vi "python analysis.vi"() -> ()   [LabVIEW 2020, in "Point Grey Camera.lvclass"]
uses:
  Point Grey Camera.lvclass
  Point Grey Camera.lvclass/Point Grey Camera.ctl
panel:
  out "analysis time":u32
  out "FakeCamera out":refnum<class "Point Grey Camera.lvclass">
  in  "FakeCamera in":refnum<class "Point Grey Camera.lvclass">
  out "error out":errorcluster
  in  "error in (no error)":errorcluster
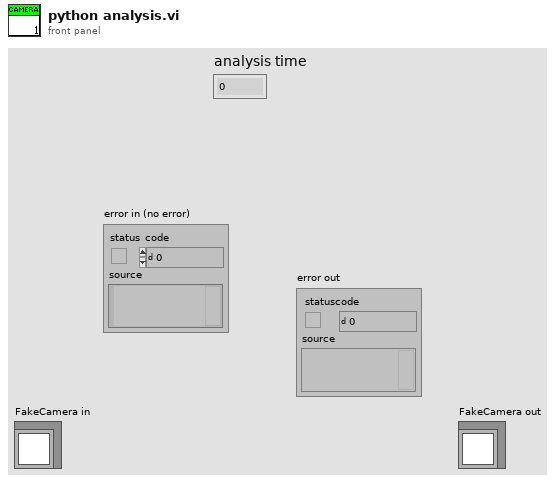
[diagram p1: front panel]
types:
  T1 = typedef "OnOffTypeDef.ctl" = enum16{"off", "on"}
  T2 = typedef "IMAQ Image.ctl" = refnum<image>
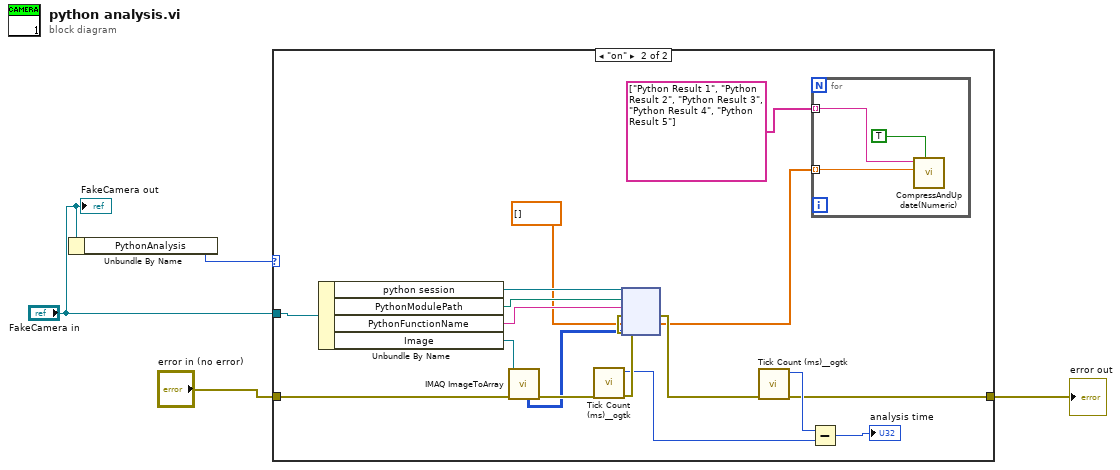
[diagram p0: block diagram]
diagram:
  n1 = Unbundle By Name("FakeCamera in") -> ("PythonAnalysis"=w1:T1)
  n2 = case shown="\"on\"" w1 {
    tunnel: "error in (no error)" -> [w5 w13]
    tunnel: [w5 w20] -> w3
    tunnel: "FakeCamera in" -> [_ w18]
    frame "off", Default {
    }
    frame "on" {
      n3 = Unbundle By Name(w18) -> ("python session"=w16:refnum<k35>, "PythonModulePath"=w15:path, "PythonFunctionName"=w14:string, "Image"=w17:T2)
      n4 = call "IMAQ ImageToArray"("error in (no error)"=w13, "Image"=w17) -> ("Image Pixels (U16)"=w8:u16[][], "error out"=w12:errorcluster)  [unwired: 2 in, 3 out]
      n5 = call "Tick Count (ms)__ogtk.vi"("error in (no error)"=w12) -> ("error out"=w11:errorcluster, "millisecond timer value"=w9:u32)  [unwired: 9 in]
      n6 = node(w16, w15, w14, w11, dbl[] [], w8) -> (w10:errorcluster, w6:dbl[])  [unwired: 1 in, 3 out]
      n7 = call "Tick Count (ms)__ogtk.vi"("error in (no error)"=w10) -> ("error out"=w20:errorcluster, "millisecond timer value"=w21:u32)  [unwired: 9 in]
      n8 = Subtract(x=w21, y=w9) -> (x-y=→"analysis time":u32)
      n9 = for {
        tunnel: string[] ["Python Result 1", "Python Result 2", "Python Result 3", "Python Result 4", "Python Result 5"] -> [w24] mode=indexing
        tunnel: w6 -> [w23] mode=indexing
        n10 = call "CompressAndUpdate(Numeric).vi"("force CVT update (false)"=TRUE, "Numeric"=w23, "command or variable name"=w24) -> ()  [unwired: 8 in, 1 out]
      }
    }
  }
  "error out" <- w3
  "FakeCamera out" <- "FakeCamera in"
